vi "Stop Core.vi"(10 "final error code":i32, 11 "Main Display in":refnum<class "Main Display.lvclass">) -> (3 "Main Display out":refnum<class "Main Display.lvclass">)   [LabVIEW 2016, in "Assert Display.lvlib" / "Main Display.lvlib" / "Main Display.lvclass"]
doc: "(<B>Filename</B>: Actor Framework.lvlib:Actor.lvclass:Stop Core.vi)\n\nDefines what the actor does before it stops. Use the <B>final error code</B> input to determine whether the actor shut down in response to an error.\n\nBy default, this method does nothing. A descendant class may override it to define behavior, such as shutting down any processes the actor initiated in its override of the Actor Core method."
uses:
  Main Display.lvclass
  Main Display.lvclass/Main Display.ctl
  <vilib>/ActorFramework/Stop Msg/Stop Msg.lvclass/Stop Msg.ctl
  <vilib>/ActorFramework/Message Enqueuer/Message Enqueuer.lvclass/Message Enqueuer.ctl
  <vilib>/ActorFramework/Stop Msg/Send Emergency Stop.vi
  <vilib>/ActorFramework/Stop Msg/Send Normal Stop.vi
  <vilib>/ActorFramework/Message Enqueuer/Enqueue Critical.vi
  <vilib>/ActorFramework/Message Enqueuer/Enqueue.vi
  <vilib>/ActorFramework/Stop Msg/Stop Msg.lvclass
  C:/Program Files (x86)/National Instruments/LabVIEW 2016/vi.lib/ActorFramework/Message/Message.lvclass
  <vilib>/ActorFramework/Message Priority Queue/Priority Enqueue.vi
  Base UI Component/Base UI Component/Base UI Component.lvclass
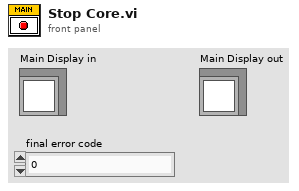
[diagram p1: front panel]
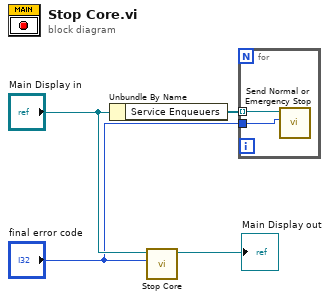
[diagram p0: block diagram]
diagram:
  n1 = Unbundle By Name("Main Display in") -> ("Service Enqueuers"=w3:refnum<class "Message Enqueuer.lvclass">[])
  n2 = call-parent "Stop Core.vi"("final error code"="final error code", "Base UI Component in"="Main Display in") -> ("Base UI Component out"=→"Main Display out":refnum<class "Main Display.lvclass">)  [unwired: 9 in]
  n3 = for {
    tunnel: w3 -> [w6] mode=indexing
    tunnel: "final error code" -> [w5]
    n4 = call <vilib>:"Send Normal or Emergency Stop.vi"("final error code"=w5, "Message Enqueuer"=w6) -> ()  [unwired: 9 in, 1 out]
  }
